vi "Create Voltage and Current graphs.vi"(8 "error in (no error)":errorcluster, 11 "Refnum in":refnum<k34>) -> (0 "error out":errorcluster, 1 "Full Shot":waveform(dbl)[](array[waveform]), 2 "Single Pulse":waveform(dbl)[](array[waveform]), 3 "Refnum out":refnum<k34>)   [LabVIEW 2015]
uses:
  <vilib>/Waveform/WDTOps.llb/WDT Get Waveform Subset DBL.vi
  <vilib>/Analysis/NI_AAL_SigProc.lvlib
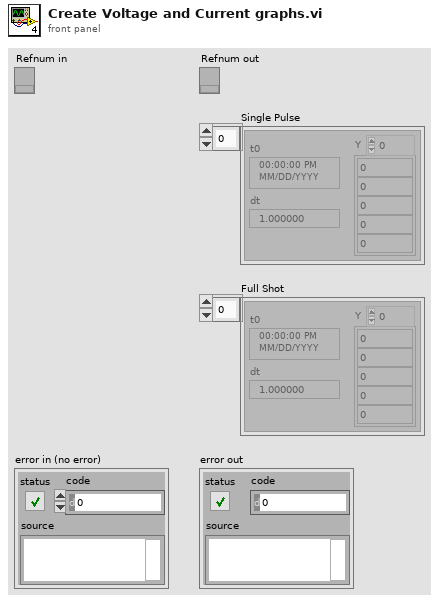
[diagram p1: front panel]
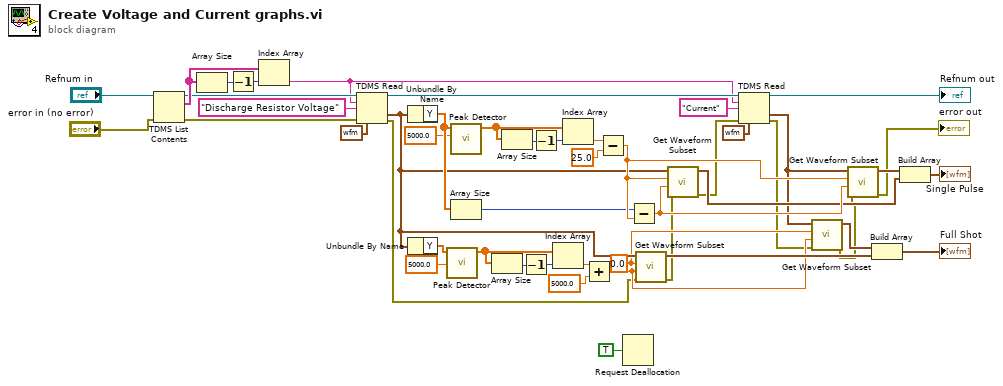
[diagram p0: block diagram]
diagram:
  w8 = 0.0 ("start samples/time")
  n1 = TDMS List Contents(4:"error in (no error)", 7:"Refnum in") -> (0:w24:errorcluster, 2:w21:string[], 3:w20:refnum<k34>)  [unwired: 1 in, 1 out]
  n2 = Array Size(array=w21) -> (size(s)=w23:i32)
  n3 = Decrement(x=w23) -> (x-1=w22:i32)
  n4 = Index Array(array=w21, index=w22) -> (element=w19:string)
  n5 = TDMS Read(0:w20, 5:w19, 7:"Discharge Resistor Voltage" ("group name in"), 11:w24, 12:waveform(dbl) {"t0"=timestamp(0 s since 1904-01-01), "dt"=1.0, "Y"=[]} ("Waveform")) -> (4:w37:refnum<k34>, 10:w15:waveform(dbl), 15:w5:errorcluster)  [unwired: 3 in, 3 out]
  n6 = Unbundle By Name(w15) -> ("Y"=w32:dbl[])
  n7 = Unbundle By Name(w15) -> ("Y"=w18:dbl[])
  n8 = call <vilib>:"Peak Detector.vi"("threshold"=5000.0, "X"=w18) -> ("Locations"=w16:dbl[])  [unwired: 5 in, 4 out]
  n9 = call <vilib>:"Peak Detector.vi"("threshold"=5000.0, "X"=w32) -> ("Locations"=w30:dbl[])  [unwired: 5 in, 4 out]
  n10 = Array Size(array=w32) -> (size(s)=w33:i32)
  n11 = Array Size(array=w16) -> (size(s)=w14:i32)
  n12 = Array Size(array=w30) -> (size(s)=w35:i32)
  n13 = Decrement(x=w14) -> (x-1=w13:i32)
  n14 = Decrement(x=w35) -> (x-1=w36:i32)
  n15 = Index Array(array=w16, index=w13) -> (element=w12:dbl)
  n16 = Index Array(array=w30, index=w36) -> (element=w34:dbl)
  n17 = Add(x=w12, y=5000.0) -> (x+y=w7:dbl)
  n18 = Subtract(x=w34, y=25.0) -> (x-y=w46:dbl)
  n19 = Request Deallocation(TRUE ("flag")) -> ()
  n20 = Subtract(x=w33, y=w46) -> (x-y=w47:dbl)
  n21 = call-poly <vilib>:"Get Waveform Subset.vi"("error in (no error)"=w5, "duration"=w7, "start samples/time"=w8, "waveform in"=w15) -> ("error out"=w4:errorcluster, "waveform out"=w9:waveform(dbl))  [unwired: 2 in, 2 out]
  n22 = call-poly <vilib>:"Get Waveform Subset.vi"("error in (no error)"=w4, "duration"=w47, "start samples/time"=w46, "waveform in"=w15) -> ("error out"=w38:errorcluster, "waveform out"=w44:waveform(dbl))  [unwired: 2 in, 2 out]
  n23 = TDMS Read(0:w37, 5:w19, 7:"Current" ("group name in"), 11:w38, 12:waveform(dbl) {"t0"=timestamp(0 s since 1904-01-01), "dt"=1.0, "Y"=[]} ("Waveform")) -> (4:→"Refnum out":refnum<k34>, 10:w10:waveform(dbl), 15:w3:errorcluster)  [unwired: 3 in, 3 out]
  n24 = call-poly <vilib>:"Get Waveform Subset.vi"("error in (no error)"=w3, "duration"=w7, "start samples/time"=w8, "waveform in"=w10) -> ("error out"=w2:errorcluster, "waveform out"=w6:waveform(dbl))  [unwired: 2 in, 2 out]
  n25 = call-poly <vilib>:"Get Waveform Subset.vi"("error in (no error)"=w2, "duration"=w47, "start samples/time"=w46, "waveform in"=w10) -> ("error out"=→"error out":errorcluster, "waveform out"=w43:waveform(dbl))  [unwired: 2 in, 2 out]
  n26 = Build Array(w6, w9) -> (→"Full Shot":waveform(dbl)[])
  n27 = Build Array(w43, w44) -> (→"Single Pulse":waveform(dbl)[])
